vi "Initialize KnownHosts.vi"(8 "Error In":errorcluster, 11 "Session In":refnum<class "Session.lvclass">) -> (0 "Error Out":errorcluster, 2 "Handle":u64, 3 "Session Out":refnum<class "Session.lvclass">)   [LabVIEW 2017, in "LabSSH2.lvlib" / "Session.lvclass"]
uses:
  Session.lvclass
  Session.lvclass/Session.ctl
  <vilib>/Utility/error.llb/Error Cluster From Error Code.vi
  <vilib>/ErrorRing/Error Ring.xnode
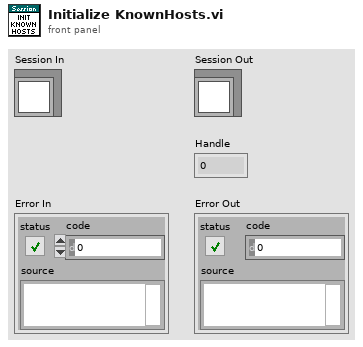
[diagram p1: front panel]
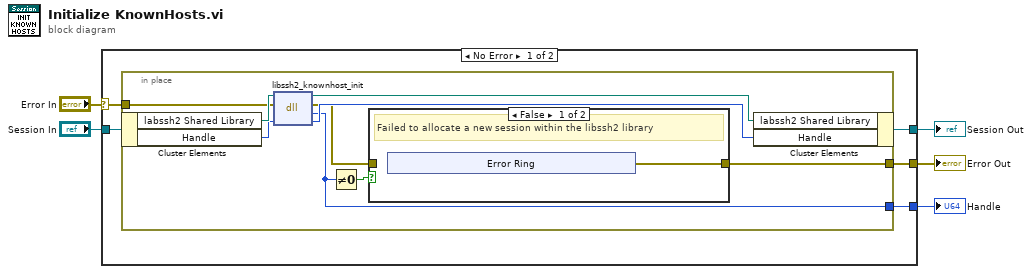
[diagram p0: block diagram]
diagram:
  n1 = case shown="No Error" "Error In" {
    selector: "Error In" -> [w8 w27]
    tunnel: [w7 w27] -> w4
    tunnel: "Session In" -> [w10 w26]
    tunnel: [w9 w26] -> w2
    tunnel: [w6 _] -> w1
    frame No Error {
      n2 = in-place {
        in-place-border: w8 -> [w17]
        in-place-border: [w13] -> w7
        in-place-border: [w11] -> w6
        n3 = in-place-cluster #1(w10) -> ("labssh2 Shared Library"=w19:path, "Handle"=w16:u64)
        n4 = dll-call lib="D:/Users/cfield/Code/Field R&D Services/SSH/LabSSH2/LabVIEW/trunk/src/LabSSH2/Private/labssh2.*" fn="libssh2_knownhost_init"(path in=w19, error in=w17, "session"=w16) -> (path out=w18:path, error out=w12:errorcluster, "KNOWNHOSTS"=w11:u64, "session"=w15:u64)  [unwired: 1 in]
        n5 = Not Equal To 0?(x=w11) -> (x != 0?=w14:bool)
        n6 = case shown="False" w14 {
          tunnel: [w20 w25] -> w13
          tunnel: w12 -> [_ w25]
          frame False {
            # "Failed to allocate a new session within the libssh2 library"
            n7 = xnode "Error Ring"() -> ("error out"=w20:errorcluster)
          }
          frame True {
            # "Success"
          }
        }
        n8 = in-place-cluster #1("labssh2 Shared Library"=w18, "Handle"=w15) -> (w9:refnum<class "Session.lvclass">)
      }
    }
    frame Error {
    }
  }
  "Error Out" <- w4
  "Session Out" <- w2
  "Handle" <- w1
